vi "Test Create.vi"() -> ()   [LabVIEW 2014, in "Arduino LiquidCrystal Wrapper.lvlib"]
uses:
  Arduino LiquidCrystal Wrapper.lvlib
panel:
  out "Error Out":errorcluster
  in  "Error In":errorcluster
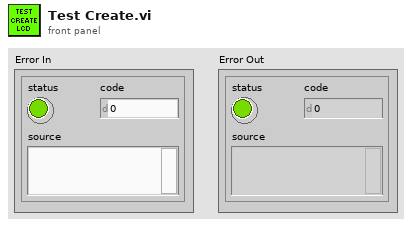
[diagram p1: front panel]
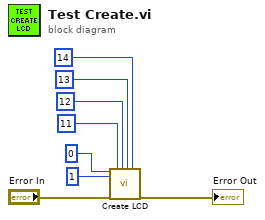
[diagram p0: block diagram]
diagram:
  n1 = call "Create LCD.vi"("rs"=u8 0, "enable"=u8 1, "Error In"="Error In", "d4"=u8 11, "d5"=u8 12, "d6"=u8 13, "d7"=u8 14) -> ("Error Out"=→"Error Out":errorcluster)  [unwired: 12 in]
